vi "Read Default Dot Cluster.vi"(8 "error in (no error)":errorcluster, 11 "Dot Settings in":refnum<class "Dot Settings.lvclass">) -> (0 "error out":errorcluster, 2 "Default Dot":T1, 3 "Dot Settings out":refnum<class "Dot Settings.lvclass">)   [LabVIEW 2019, in "Dot Settings.lvclass"]
uses:
  Dot Settings.lvclass
  TypeDefs/Default Dot Cluster.ctl
  TypeDefs/Action.ctl
  Dot Settings.lvclass/Dot Settings.ctl
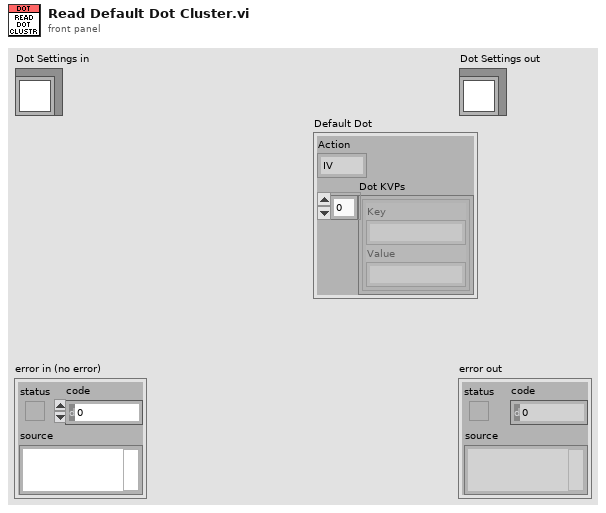
[diagram p1: front panel]
types:
  T1 = typedef "Dot Settings.lvclass/Default Dot Cluster.ctl" = cluster{"Action":T2, "Dot KVPs":cluster{"Key":string, "Value":string}[]}
  T2 = typedef "Dot Settings.lvclass/Action.ctl" = enum16{"IV", "QD"}
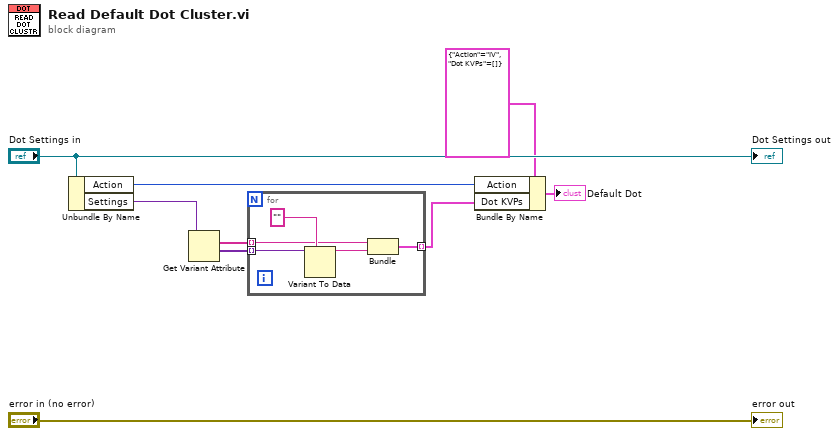
[diagram p0: block diagram]
diagram:
  n1 = Unbundle By Name("Dot Settings in") -> ("Action"=w7:T2, "Settings"=w6:variant)
  n2 = Get Variant Attribute(Variant=w6) -> (names=w5:string[], values=w4:variant[])  [unwired: 3 in, 2 out]
  n3 = for {
    tunnel: w5 -> [w11] mode=indexing
    tunnel: w4 -> [w14] mode=indexing
    tunnel: [w10] -> w3 mode=indexing
    n4 = Variant To Data(type="", Variant=w14) -> (data=w12:string)  [unwired: 1 in, 1 out]
    n5 = Bundle(w11, w12) -> (w10:cluster{string, string})  [unwired: 1 in]
  }
  n6 = Bundle By Name(cluster=T1 {"Action"=enum."IV", "Dot KVPs"=[]}, "Action"=w7, "Dot KVPs"=w3) -> (→"Default Dot":T1)
  "error out" <- "error in (no error)"
  "Dot Settings out" <- "Dot Settings in"
